vi "read_IMU_two_datasets.vi"(3 "error in (no error)":errorcluster, 4 "Next Measurement Type":u16(ring)=5 items=["PAGE-ID"=0, "SYS_E_FLAG"=2048, "DIAG_STS"=2560, "ALM_STS"=3072, "TEMP_OUT"=3584, "X_GYRO_OUT"=4608, "Y_GYRO_OUT"=5632, "Z_GYRO_OUT"=6656, "X_ACCL_OUT"=7680, "Y_ACCL_OUT"=8704, "Z_ACCL_OUT"=9728, "X_MAGN_OUT"=10240, "Y_MAGN_OUT"=10752, "Z_MAGN_OUT"=11264, "BAROM_OUT"=12288, "X_DELTAANG_OUT"=16896, "Y_DELTAANG_OUT"=17920, "Z_DELTAANG_OUT"=18944, "X_DELTAVEL_OUT"=19968, "Y_DELTAVEL_OUT"=20992, "Z_DELTAVEL_OUT"=22016], 5 "First Measurement Type":u16(ring)=5 items=["PAGE-ID"=0, "SYS_E_FLAG"=2048, "DIAG_STS"=2560, "ALM_STS"=3072, "TEMP_OUT"=3584, "X_GYRO_OUT"=4608, "Y_GYRO_OUT"=5632, "Z_GYRO_OUT"=6656, "X_ACCL_OUT"=7680, "Y_ACCL_OUT"=8704, "Z_ACCL_OUT"=9728, "X_MAGN_OUT"=10240, "Y_MAGN_OUT"=10752, "Z_MAGN_OUT"=11264, "BAROM_OUT"=12288, "X_DELTAANG_OUT"=16896, "Y_DELTAANG_OUT"=17920, "Z_DELTAANG_OUT"=18944, "X_DELTAVEL_OUT"=19968, "Y_DELTAVEL_OUT"=20992, "Z_DELTAVEL_OUT"=22016]) -> (0 "error out":errorcluster, 1 "Last Dataset":i16, 2 "1st Dataset":i16)   [LabVIEW 2013]
uses:
  <vilib>/myRIO/Instrument Drivers/Onboard IO/DIO/vis/Smart Open.vi
  <vilib>/myRIO/Instrument Drivers/Onboard IO/DIO/vis/Write.vi
  <vilib>/myRIO/Instrument Drivers/Onboard IO/SPI/vis/Smart Open.vi
  <vilib>/myRIO/Instrument Drivers/Onboard IO/SPI/vis/Configure.vi
  <vilib>/myRIO/Instrument Drivers/Onboard IO/SPI/vis/Write Read.vi
  <vilib>/myRIO/Instrument Drivers/Onboard IO/DIO/vis/Open.vi
  <vilib>/myRIO/Instrument Drivers/Onboard IO/SPI/vis/Open.vi
  <vilib>/myRIO/Common/Instrument Driver Framework/myRIO v1.0/DIO/vis/myRIO v1.1 Open DIO.vi
  <vilib>/myRIO/Common/Instrument Driver Framework/myRIO v1.0/SPI/vis/myRIO v1.1 Open SPI.vi
  <vilib>/myRIO/Common/Instrument Driver Framework/Utilities/vis/Validate Channels.vi
  <vilib>/myRIO/Common/Instrument Driver Framework/myRIO v1.0/DIO/vis/myRIO v1.0 Reserve DIO.vi
  <vilib>/myRIO/Common/Instrument Driver Framework/myRIO v1.0/SPI/vis/myRIO v1.0 Reserve SPI.vi
  <vilib>/myRIO/Common/Instrument Driver Framework/myRIO v1.0/Resource Manager/vis/myRIO v1.0 Reserve Channel List.vi
  <vilib>/myRIO/Common/Instrument Driver Framework/myRIO v1.0/DIO/vis/myRIO v1.0 Build MUX Configuration DIO.vi
  <vilib>/myRIO/Common/Instrument Driver Framework/myRIO v1.0/SPI/vis/myRIO v1.0 Build MUX Configuration SPI.vi
  <vilib>/myRIO/Common/Instrument Driver Framework/myRIO v1.0/Resource Manager/vis/myRIO v1.0 Reserve Channel.vi
  <vilib>/myRIO/Common/Instrument Driver Framework/myRIO v1.0/Resource Manager/vis/myRIO v1.0 Unreserve Channel.vi
  <vilib>/myRIO/Common/Instrument Driver Framework/myRIO v1.0/Resource Manager/vis/myRIO v1.0 Create Configuration List.vi
  <vilib>/myRIO/Common/Instrument Driver Framework/myRIO v1.0/Resource Manager/vis/myRIO v1.0 Build Mutex Name.vi
  <vilib>/myRIO/Common/Instrument Driver Framework/myRIO v1.0/myRIO v1.1 Open.vi
  <vilib>/Utility/VariantDataType/GetNumericInfo.vi
  <vilib>/Utility/error.llb/Error Cluster From Error Code.vi
  <vilib>/myRIO/Common/Instrument Driver Framework/Utilities/vis/IO Manager.vi
  <vilib>/myRIO/Common/Instrument Driver Framework/Utilities/vis/Configuration Manager.vi
  <vilib>/myRIO/Common/Instrument Driver Framework/myRIO v1.0/Resource Manager/vis/myRIO v1.0 Configure IO.vi
  <vilib>/myRIO/Common/Instrument Driver Framework/myRIO v1.0/myRIO v1.0 Close.vi
  <vilib>/myRIO/Common/Instrument Driver Framework/myRIO v1.0/DIO/vis/myRIO v1.0 Write DIO.vi
  <vilib>/myRIO/Common/Instrument Driver Framework/myRIO v1.0/SPI/vis/myRIO v1.0 Configure SPI.vi
  <vilib>/myRIO/Common/Instrument Driver Framework/myRIO v1.0/SPI/vis/myRIO v1.0 Write Read SPI.vi
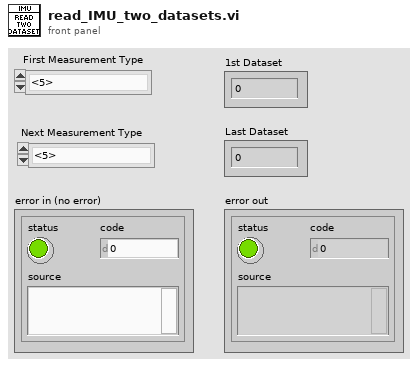
[diagram p1: front panel]
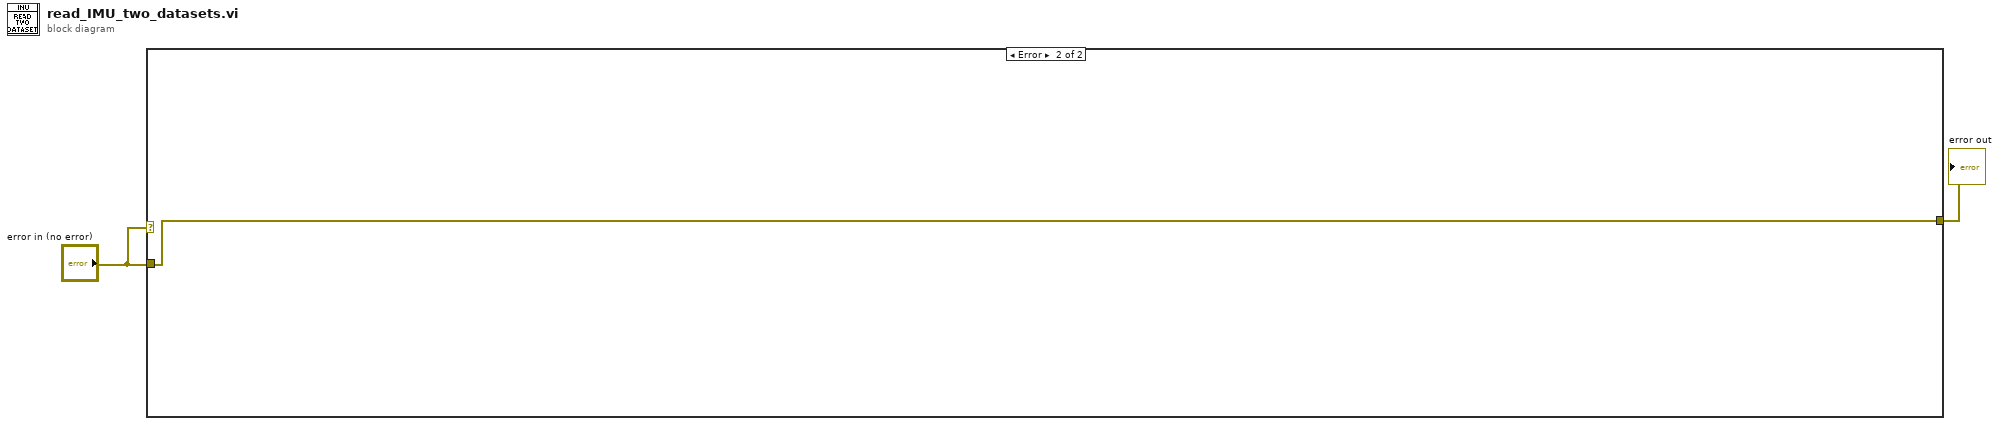
[diagram p0: block diagram]
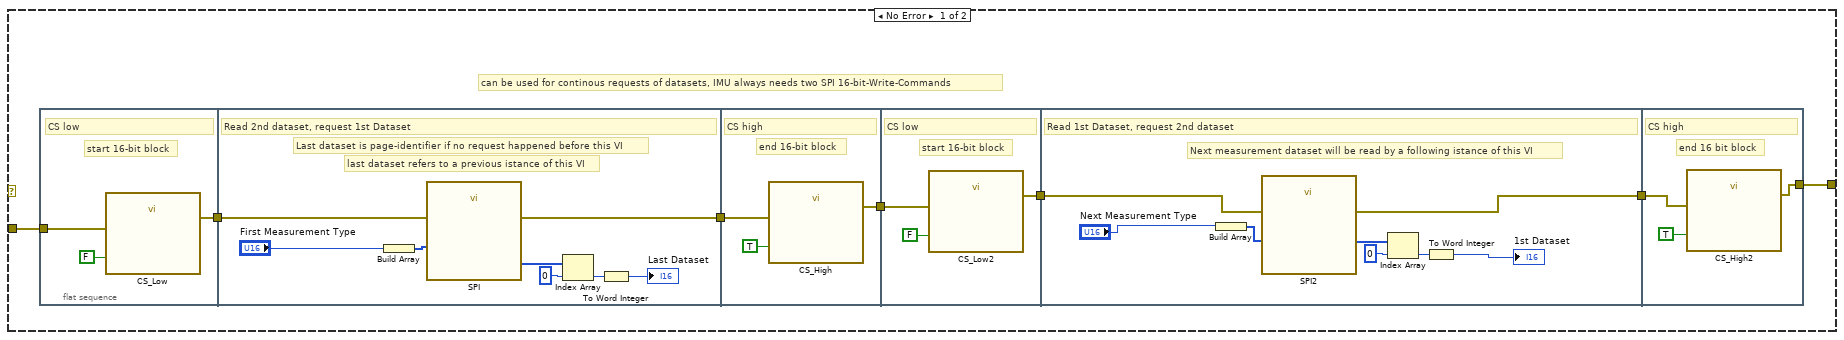
[diagram p2: hidden frame]
diagram:
  n1 = case shown="Error" "error in (no error)" {
    tunnel: "error in (no error)" -> [w4 w38]
    tunnel: [w3 w38] -> w2
    frame No Error {
      # "can be used for continous requests of datasets, IMU always needs two SPI 16-bit-Write-Commands"
      n2 = flat-sequence {
        tunnel: [w10] -> w9
        tunnel: w4 -> [w11]
        tunnel: w9 -> [w20]
        tunnel: [w18] -> w8
        tunnel: [w21] -> w7
        tunnel: w8 -> [w22]
        tunnel: [w24] -> w6
        tunnel: w7 -> [w26]
        tunnel: w6 -> [w32]
        tunnel: [w30] -> w5
        tunnel: [w35] -> w3
        tunnel: w5 -> [w36]
        frame #0 {
          # "start 16-bit block"
          # "CS low"
          n3 = call "CS_Low"("Slave_select_IMU (A/DIO4 (Pin 19))"=FALSE, "error in (no error)"=w11) -> ("error out"=w10:errorcluster)  [unwired: 25 in]
        }
        frame #1 {
          # "last dataset refers to a previous istance of this VI"
          # "Last dataset is page-identifier if no request happened before this VI"
          # "Read 2nd dataset, request 1st Dataset"
          n4 = Build Array("First Measurement Type") -> (w19:u16[])
          n5 = call "SPI"("Frames to Write"=w19, "error in (no error)"=w20) -> ("Frames Read"=w15:u16[], "error out"=w18:errorcluster)  [unwired: 24 in]
          n6 = Index Array(array=w15, index=0) -> (element=w17:u16)
          n7 = To Word Integer(number=w17) -> (16bit integer=→"Last Dataset":i16)
        }
        frame #2 {
          # "end 16-bit block"
          # "CS high"
          n8 = call "CS_High"("Slave_select_IMU (A/DIO4 (Pin 19))"=TRUE, "error in (no error)"=w22) -> ("error out"=w21:errorcluster)  [unwired: 25 in]
        }
        frame #3 {
          # "start 16-bit block"
          # "CS low"
          n9 = call "CS_Low2"("Slave_select_IMU (A/DIO4 (Pin 19))"=FALSE, "error in (no error)"=w26) -> ("error out"=w24:errorcluster)  [unwired: 25 in]
        }
        frame #4 {
          # "Next measurement dataset will be read by a following istance of this VI"
          # "Read 1st Dataset, request 2nd dataset"
          n10 = Build Array("Next Measurement Type") -> (w31:u16[])
          n11 = call "SPI2"("Frames to Write"=w31, "error in (no error)"=w32) -> ("Frames Read"=w33:u16[], "error out"=w30:errorcluster)  [unwired: 24 in]
          n12 = Index Array(array=w33, index=0) -> (element=w29:u16)
          n13 = To Word Integer(number=w29) -> (16bit integer=→"1st Dataset":i16)
        }
        frame #5 {
          # "end 16 bit block"
          # "CS high"
          n14 = call "CS_High2"("Slave_select_IMU (A/DIO4 (Pin 19))"=TRUE, "error in (no error)"=w36) -> ("error out"=w35:errorcluster)  [unwired: 25 in]
        }
      }
    }
    frame Error {
    }
  }
  "error out" <- w2
